vi "Fire Connect Event.vi"(6 "Mux Index":i32, 8 "error in (no error)":errorcluster, 9 "Output":i32, 10 "Input":i32, 11 "MuxPanel in":refnum<class "MuxPanel.lvclass">) -> (0 "error out":errorcluster, 3 "MuxPanel out":refnum<class "MuxPanel.lvclass">)   [LabVIEW 2022 SP3, in "TouchControl.lvlib" / "MuxPanel.lvclass"]
uses:
  MuxPanel.lvclass
  MuxPanel.lvclass/MuxPanel.ctl
  Connection.ctl
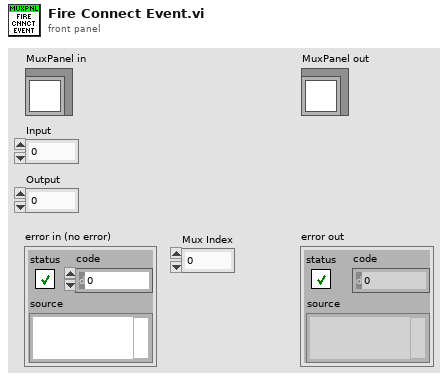
[diagram p1: front panel]
types:
  T1 = typedef "TouchControl.lvlib/MuxPanel.lvclass/Connection.ctl" = cluster{"Mux Index":i32, "Input":i32, "Output":i32}
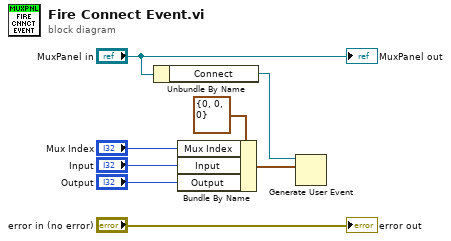
[diagram p0: block diagram]
diagram:
  n1 = Unbundle By Name("MuxPanel in") -> ("Connect"=w6:refnum<user-event>)
  n2 = Bundle By Name(cluster=T1 {"Mux Index"=0, "Input"=0, "Output"=0} ("event data"), "Mux Index"="Mux Index", "Input"="Input", "Output"="Output") -> (w4:T1)
  n3 = Generate User Event(user event=w6, event data cluster=w4) -> ()  [unwired: 2 in, 2 out]
  "error out" <- "error in (no error)"
  "MuxPanel out" <- "MuxPanel in"
